vi "Remove Invalid File Characters.vi"(11 "String In":string) -> (3 "String Out":string)   [LabVIEW 2013]
uses:
  <vilib>/regexp/Match Regular Expression.xnode
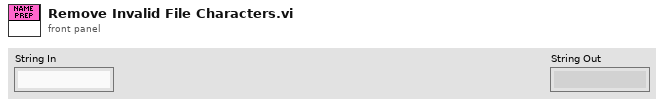
[diagram p1: front panel]
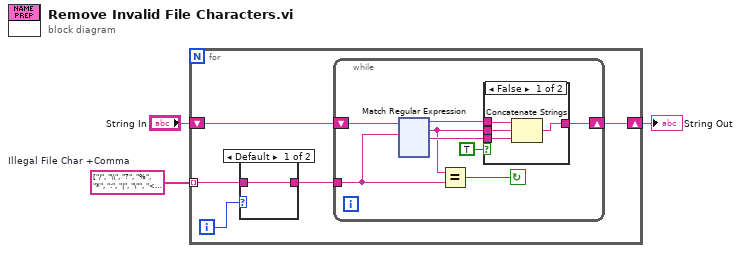
[diagram p0: block diagram]
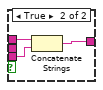
[diagram p3: hidden frame]
diagram:
  w3 = string[] ["/", "\\", "?", "%", "*", ":", "|", "\"", "<", ">", "[.]", ","]  # Illegal File Char +Comma
  n1 = for {
    shift-right: [w7] -> w1
    shift-left: "String In" -> [w8]
    tunnel: w3 -> [w5] mode=indexing
    i -> [w6]
    n2 = case shown="Default" w6 {
      tunnel: w5 -> [w9 w10]
      tunnel: [w9 w10] -> w4
      frame Default {
      }
      frame 10 {
      }
    }
    n3 = while {
      tunnel: w4 -> [w15]
      shift-right: [w12] -> w7
      shift-left: w8 -> [w18]
      stop <- w14 continue-if-true
      n4 = xnode "Match Regular Expression"("input string"=w18, "regular expression"=w15) -> ("before match"=w17:string, "whole match"=w13:string, "after match"=w16:string)  [unwired: 4 in, 2 out]
      n5 = Equal?(x=w13, y=w15) -> (x = y?=w14:bool)
      n6 = case shown="False" TRUE {
        tunnel: w17 -> [w21 w25]
        tunnel: w16 -> [w22 w24]
        tunnel: [w20 w23] -> w12
        tunnel: w13 -> [w19 _]
        frame False {
          n7 = Concatenate Strings(w21, w19, w22) -> (w20:string)
        }
        frame True {
          n8 = Concatenate Strings(w25, w24) -> (w23:string)
        }
      }
    }
  }
  "String Out" <- w1
